vi "amc_Update Message Routing Info.vi"(4 "Source Process":string, 5 "Acknowledge Message (F)":bool, 6 "Source Host":string, 7 "Priority Message (F)":bool, 9 "Receiver Process":string, 10 "Receiver Host":string, 11 "Message":T1) -> (3 "Message":T1)   [LabVIEW 2012, in "REx_Springboard.lvlib" / "TLB_Dependencies.lvlib"]
uses:
  TLB_Dependencies.lvlib
  amc_Message.ctl
  <vilib>/FTP/util/Keyed Array.ctl
  <vilib>/FTP/NI_FTP.lvlib
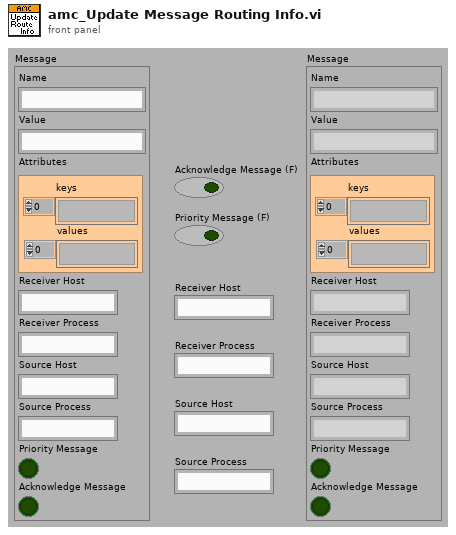
[diagram p1: front panel]
types:
  T1 = typedef "REx_Springboard.lvlib/TLB_Dependencies.lvlib/amc_Message.ctl" = cluster{"Name":string, "Value":string, "Attributes":T2, "Receiver Host":string, "Receiver Process":string, "Source Host":string, "Source Process":string, "Priority Message":bool, "Acknowledge Message":bool}
  T2 = typedef "NI_FTP.lvlib/Keyed Array.ctl" = cluster{"keys":string[], "values":string[]}
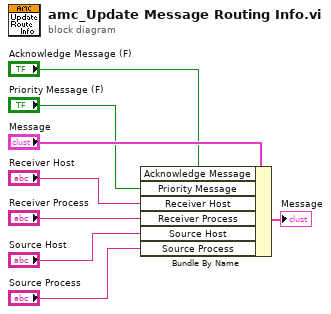
[diagram p0: block diagram]
diagram:
  n1 = Bundle By Name(cluster="Message", "Acknowledge Message"="Acknowledge Message (F)", "Priority Message"="Priority Message (F)", "Receiver Host"="Receiver Host", "Receiver Process"="Receiver Process", "Source Host"="Source Host", "Source Process"="Source Process") -> (→"Message":T1)
